vi "Viewing Distance.vi"(10 "Tree":u8, 11 "Trees":u8[](array[numeric])) -> (3 "NTrees":i64)   [LabVIEW 2021, in "d8.lvlib"]
uses:
  d8.lvlib
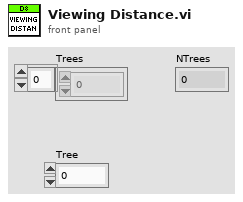
[diagram p1: front panel]
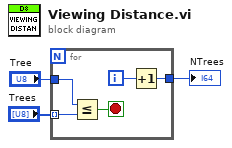
[diagram p0: block diagram]
diagram:
  n1 = for {
    tunnel: "Tree" -> [w8]
    tunnel: "Trees" -> [w7] mode=indexing
    tunnel: [w4] -> w1
    i -> [w5]
    stop <- w6 stop-if-true
    n2 = Less Or Equal?(x=w8, y=w7) -> (x <= y?=w6:bool)
    n3 = Increment(x=w5) -> (x+1=w4:i32)
  }
  "NTrees" <- w1
